vi "read_T.vi"(7 "Enum":T1(ring), 8 "error in":errorcluster, 10 "physical channels":tag) -> (0 "error out":errorcluster, 2 "data":dbl[](array[numeric]) format="%0.2f")   [LabVIEW 2015]
uses:
  <vilib>/DAQmx/read.llb/DAQmx Read (Analog 1D Wfm NChan NSamp).vi
  <vilib>/Analysis/5stat.llb/RMS (DBL).vi
  <vilib>/DAQmx/create/channels.llb/DAQmx Create Channel (AI-Voltage-Basic).vi
  <vilib>/DAQmx/configure/timing.llb/DAQmx Timing (Sample Clock).vi
  <vilib>/DAQmx/miscellaneous.llb/DAQmx Fill In Error Info.vi
  <vilib>/Analysis/NI_AALPro.lvlib
panel:
  out "error out 2":errorcluster
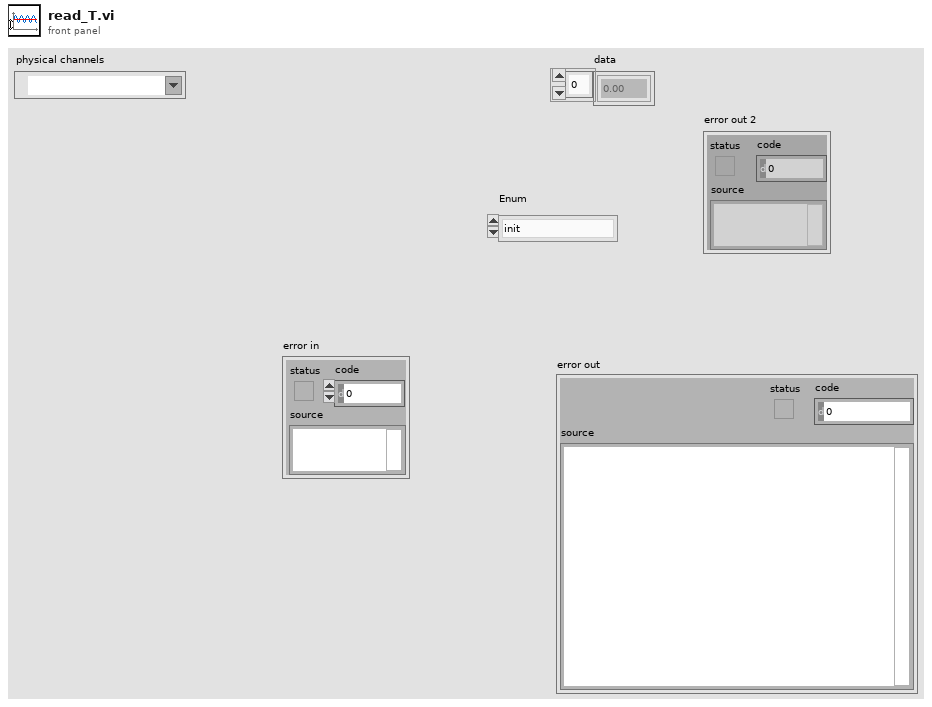
[diagram p1: front panel]
types:
  T1 = enum16{"init", "config", "start", "read", "stop"}
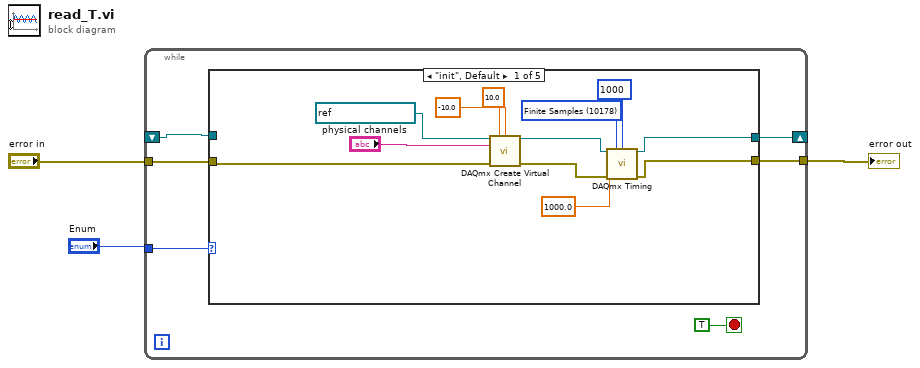
[diagram p0: block diagram]
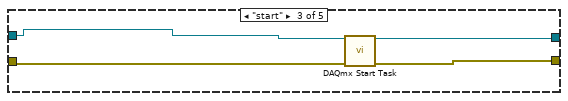
[diagram p3: hidden frame]
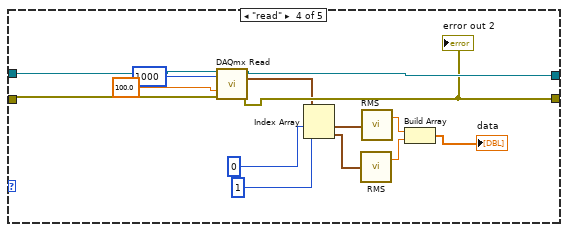
[diagram p4: hidden frame]
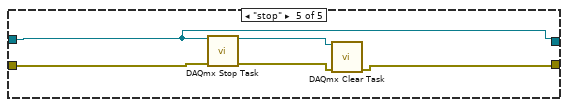
[diagram p5: hidden frame]
diagram:
  n1 = while {
    tunnel: "Enum" -> [w8]
    shift-right: [w7] -> _
    shift-left: _ -> [w6]
    tunnel: "error in" -> [w5]
    tunnel: [w4] -> w1
    stop <- TRUE stop-if-true
    n2 = case shown="\"init\", Default" w8 {
      tunnel: [w18 w22 w27 w39 w42] -> w7
      tunnel: w6 -> [_ w22 w25 w41 w42]
      tunnel: w5 -> [w21 w23 w24 w40 w46]
      tunnel: [w15 w23 w26 w38 w45] -> w4
      frame "init", Default {
        w13 = 10178 items=["Finite Samples"=10178, "Continuous Samples"=10123, "Hardware Timed Single Point"=12522] ("sample mode")
        n3 = call-poly <vilib>:"DAQmx Create Virtual Channel.vi"("task in"=refnum<k21> "我的电压任务", "maximum value"=10.0, "minimum value"=-10.0, "physical channels"="physical channels", "error in"=w21) -> ("task out"=w19:refnum<k21>, "error out"=w16:errorcluster)  [unwired: 9 in]
        n4 = call-poly <vilib>:"DAQmx Timing.vi"("task/channels in"=w19, "sample mode"=w13, "samples per channel"=1000, "rate"=1000.0, "error in"=w16) -> ("task out"=w18:refnum<k21>, "error out"=w15:errorcluster)  [unwired: 9 in]
      }
      frame "config" {
      }
      frame "start" {
        n5 = call <vilib>:"DAQmx Start Task.vi"("task/channels in"=w25, "error in"=w24) -> ("task out"=w27:refnum<k21>, "error out"=w26:errorcluster)  [unwired: 12 in]
      }
      frame "read" {
        n6 = call-poly <vilib>:"DAQmx Read.vi"("task/channels in"=w41, "number of samples per channel"=1000, "timeout"=100.0, "error in"=w40) -> ("task out"=w39:refnum<k21>, "data"=w35:waveform(dbl)[], "error out"=w38:errorcluster)  [unwired: 9 in]
        "error out 2" <- w38
        n7 = Index Array(array=w35, index #1=0 ("index"), index #2=1 ("index")) -> (element #1=w32:waveform(dbl), element #2=w31:waveform(dbl))
        n8 = call-poly <vilib>:"RMS.vi"("X"=w31) -> ("rms value"=w29:dbl)  [unwired: 1 out]
        n9 = call-poly <vilib>:"RMS.vi"("X"=w32) -> ("rms value"=w30:dbl)  [unwired: 1 out]
        n10 = Build Array(w30, w29) -> (→"data":dbl[])
      }
      frame "stop" {
        n11 = call <vilib>:"DAQmx Stop Task.vi"("task/channels in"=w42, "error in"=w46) -> ("task out"=w44:refnum<k21>, "error out"=w43:errorcluster)  [unwired: 12 in]
        n12 = call <vilib>:"DAQmx Clear Task.vi"("task in"=w44, "error in"=w43) -> ("error out"=w45:errorcluster)  [unwired: 13 in]
      }
    }
  }
  "error out" <- w1
